vi "Solve2.vi"(8 "Error In":errorcluster, 11 "object in":refnum<class "2021_3.lvclass">) -> (0 "Error Out":errorcluster, 2 "Result":u64, 3 "object out":refnum<class "2021_3.lvclass">)   [LabVIEW 2020, in "2021_3.lvclass"]
uses:
  2021_3.lvclass
  2021_3.lvclass/2021_3.ctl
  3f4102ff-a07f-44b2-928f-cc4d439d426a.vi
  41fa4204-0662-4100-8351-9a46fc30aec6.vi
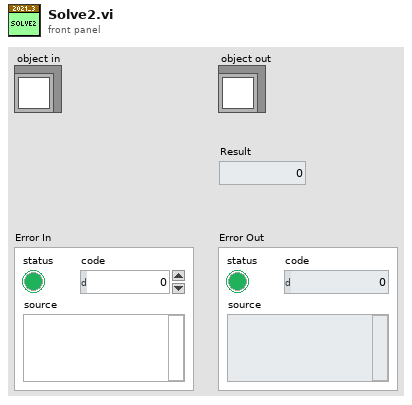
[diagram p1: front panel]
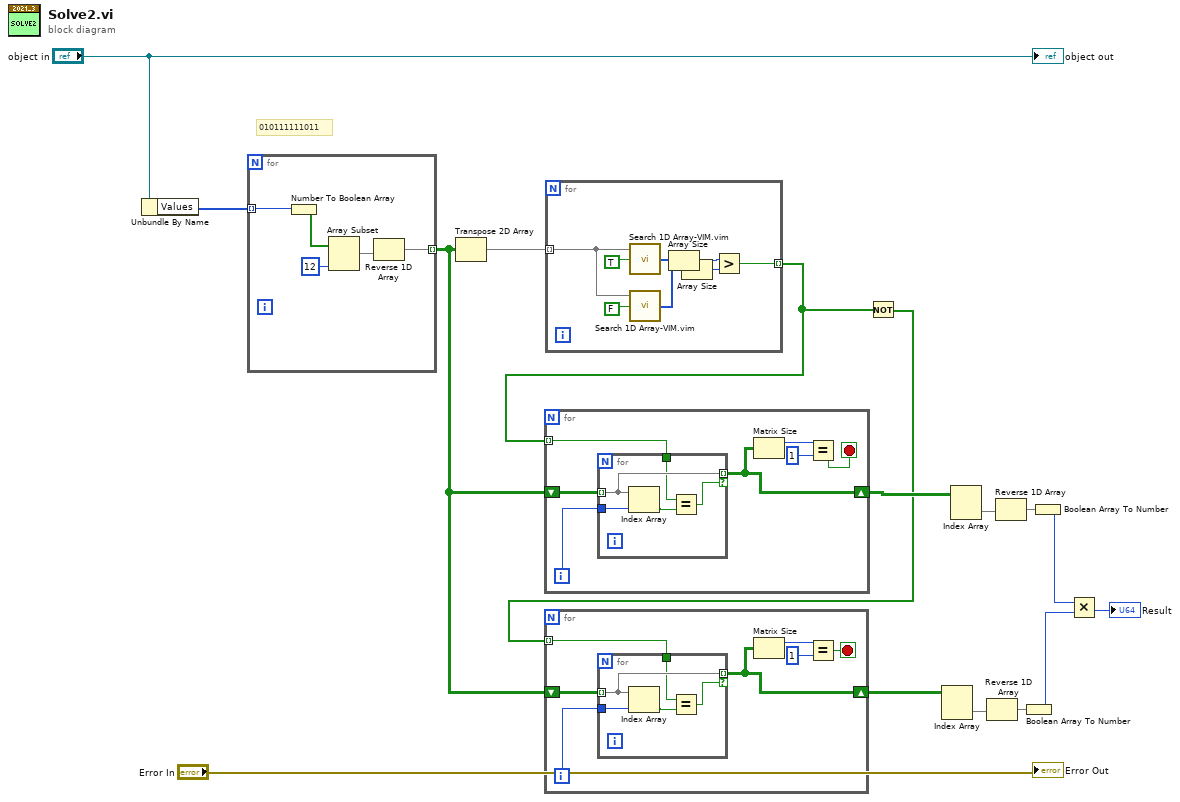
[diagram p0: block diagram]
diagram:
  # "010111111011"
  n1 = Unbundle By Name("object in") -> ("Values"=w15:u32[])
  n2 = for {
    tunnel: w15 -> [w21] mode=indexing
    tunnel: [w17] -> w5 mode=indexing
    n3 = Number To Boolean Array(number=w21) -> (Boolean array=w20:bool[])
    n4 = Array Subset(array=w20, length=12) -> (w18:bool[])  [unwired: 1 in]
    n5 = Reverse 1D Array(array=w18) -> (reversed array=w17:bool[])
  }
  n6 = Transpose 2D Array(2D array=w5) -> (transposed array=w13:bool[][])
  n7 = for {
    tunnel: w13 -> [w28] mode=indexing
    tunnel: [w22] -> w1 mode=indexing
    n8 = call "Search 1D Array-VIM.vim"("Array"=w28, "Element Data"=TRUE) -> ("Indices of Elements"=w26:i32[])  [unwired: 7 in]
    n9 = call "Search 1D Array-VIM.vim"("Array"=w28, "Element Data"=FALSE) -> ("Indices of Elements"=w25:i32[])  [unwired: 7 in]
    n10 = Array Size(array=w26) -> (size(s)=w24:i32)
    n11 = Array Size(array=w25) -> (size(s)=w23:i32)
    n12 = Greater?(x=w24, y=w23) -> (0:w22:bool)
  }
  n13 = for {
    tunnel: w1 -> [w34] mode=indexing
    shift-right: [w33] -> w12
    shift-left: w5 -> [w36]
    i -> [w35]
    stop <- w30 stop-if-true
    n14 = for {
      tunnel: w36 -> [w41] mode=indexing
      tunnel: w35 -> [w40]
      tunnel: [w41] -> w33 mode=indexing if=w37
      tunnel: w34 -> [w39]
      n15 = Index Array(array=w41, index=w40) -> (element=w38:bool)
      n16 = Equal?(x=w39, y=w38) -> (x = y?=w37:bool)
    }
    n17 = Matrix Size(0:w33) -> (1:w32:i32)  [unwired: 1 out]
    n18 = Equal?(x=w32, y=1) -> (x = y?=w30:bool)
  }
  n19 = Not(x=w1) -> (.not. x?=w6:bool[])
  n20 = for {
    tunnel: w6 -> [w46] mode=indexing
    shift-right: [w45] -> w7
    shift-left: w5 -> [w48]
    i -> [w47]
    stop <- w42 stop-if-true
    n21 = for {
      tunnel: w48 -> [w53] mode=indexing
      tunnel: w47 -> [w52]
      tunnel: [w53] -> w45 mode=indexing if=w49
      tunnel: w46 -> [w51]
      n22 = Index Array(array=w53, index=w52) -> (element=w50:bool)
      n23 = Equal?(x=w51, y=w50) -> (x = y?=w49:bool)
    }
    n24 = Matrix Size(0:w45) -> (1:w44:i32)  [unwired: 1 out]
    n25 = Equal?(x=w44, y=1) -> (x = y?=w42:bool)
  }
  n26 = Index Array(array=w7) -> (element=w8:bool[])  [unwired: 2 in]
  n27 = Index Array(array=w12) -> (element=w11:bool[])  [unwired: 2 in]
  n28 = Reverse 1D Array(array=w8) -> (reversed array=w9:bool[])
  n29 = Reverse 1D Array(array=w11) -> (reversed array=w10:bool[])
  n30 = Boolean Array To Number(Boolean array=w9) -> (number=w3:u32)
  n31 = Boolean Array To Number(Boolean array=w10) -> (number=w4:u32)
  n32 = Multiply(x=w4, y=w3) -> (x*y=→"Result":u32)
  "Error Out" <- "Error In"
  "object out" <- "object in"
